vi "Update DI DAQ IO Data.vi"(8 "error in (no error)":errorcluster, 9 "DIO in":bool[](array[boolean]), 10 "DIO ClusterArray":T2[](array[typedef]), 11 "dCVT DAQDict":T1) -> (0 "error out":errorcluster, 2 "DIO ClusterArray out":T2[](array[typedef]), 3 "dCVT DAQDict out":T1)   [LabVIEW 2020, in "DAQDict.lvlib"]
uses:
  DAQDict.lvlib
  support/IO Task--cluster.ctl
  support/IO Task Dict Node--cluster.ctl
  support/IONameNode--cluster.ctl
  support/DIO ClusterArray Element--cluster.ctl
  <vilib>/TELLC/Dynamic CVT API/TD Dynamic CVT DVR--ref.ctl
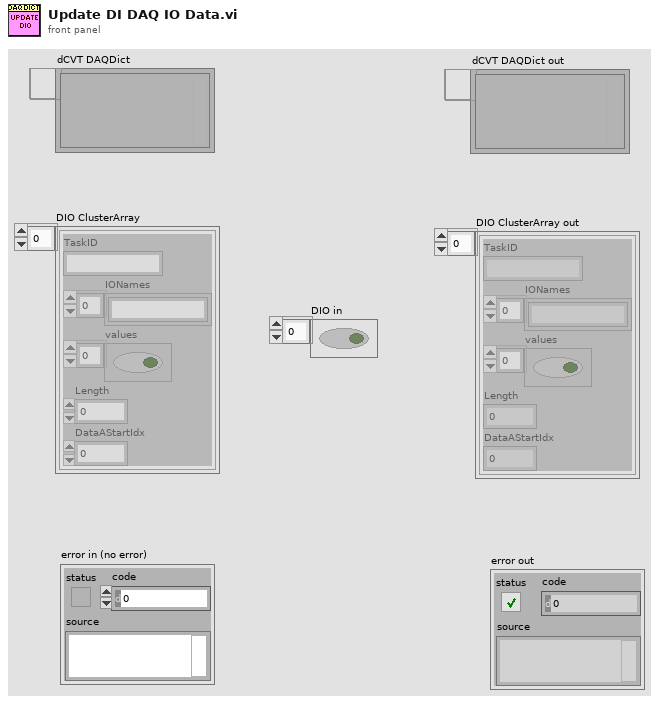
[diagram p1: front panel]
types:
  T1 = typedef "TD Dynamic CVT DVR--ref.ctl" = refnum<data-value>
  T2 = typedef "DIO ClusterArray Element--cluster.ctl" = cluster{"TaskID":string, "IONames":string[], "values":bool[], "Length":i32, "DataAStartIdx":i32}
  T3 = typedef "IO Task Dict Node--cluster.ctl" = cluster{"IO Type":enum16{"N/A", "DI", "DO"}, "IONames":string[], "values":bool[], "IO Task":T4}
  T4 = typedef "IO Task--cluster.ctl" = cluster{"IO Type":enum16{"N/A", "DI", "DO"}, "TaskID":string, "IONames":string[], "ChPath":string[], "Task Ref":refnum<k21>}
  T5 = typedef "IONameNode--cluster.ctl" = cluster{"IOName":string, "value":bool, "IO Type":enum16{"N/A", "DI", "DO"}, "TaskID":string, "data Idx":i32}
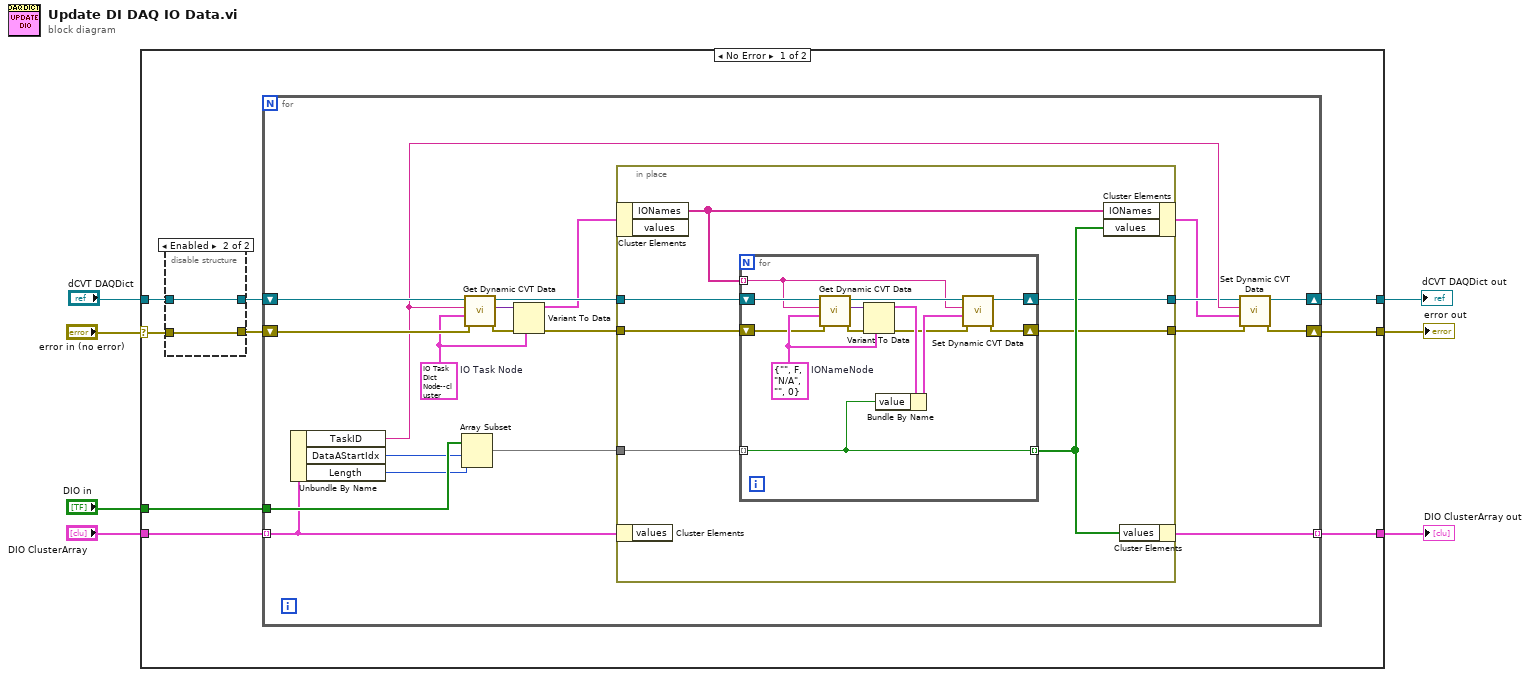
[diagram p0: block diagram]
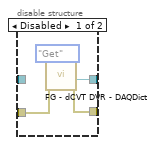
[diagram p2: hidden frame]
diagram:
  n1 = case shown="No Error" "error in (no error)" {
    selector: "error in (no error)" -> [w10 w65]
    tunnel: "DIO ClusterArray" -> [w15 w64]
    tunnel: "DIO in" -> [w14 _]
    tunnel: [w13 w64] -> w5
    tunnel: [w12 w65] -> w4
    tunnel: "dCVT DAQDict" -> [w9 w63]
    tunnel: [w8 w63] -> w1
    frame No Error {
      n2 = disable-structure shown="Enabled" {
        disable-tunnel: [w19 w22] -> w16
        disable-tunnel: [w18 w21] -> w11
        disable-tunnel: w10 -> [w17 w21]
        disable-tunnel: w9 -> [_ w22]
        frame Disabled {
          n3 = call "FG - dCVT DVR - DAQDict.vi"("error in (no error)"=w17, "Action (Get)"=enum16{"Init", "Get", "Set"}."Get") -> ("dCVT DAQDict out"=w19:T1, "error out"=w18:errorcluster)  [unwired: 7 in]
        }
        frame Enabled {
        }
      }
      n4 = for {
        shift-right: [w40] -> w8
        shift-left: w16 -> [w42]
        shift-right: [w39] -> w12
        shift-left: w11 -> [w41]
        tunnel: w15 -> [w37] mode=indexing
        tunnel: w14 -> [w38]
        tunnel: [w33] -> w13 mode=indexing
        w29 = T3 {"IO Type"=enum."N/A", "IONames"=[], "values"=[], "IO Task"={"IO Type"=enum."N/A", "TaskID"="", "IONames"=[], "ChPath"=[], "Task Ref"=""}}  # IO Task Node
        n5 = Unbundle By Name(w37) -> ("TaskID"=w36:string, "DataAStartIdx"=w35:i32, "Length"=w34:i32)
        n6 = Array Subset(array=w38, index=w35, length=w34) -> (w27:bool[])
        n7 = call <vilib>:"Get Dynamic CVT Data.vi"("error in (no error)"=w41, "default value (empty variant)"=w29, "DataName"=w36, "dCVT DVR"=w42) -> ("error out"=w31:errorcluster, "value"=w32:variant, "dCVT DVR out"=w30:T1)  [unwired: 4 in, 1 out]
        n8 = Variant To Data(error in=w31, type=w29, Variant=w32) -> (data=w28:T3, error out=w26:errorcluster)
        n9 = in-place {
          in-place-border: w30 -> [w49]
          in-place-border: w27 -> [w47]
          in-place-border: w26 -> [w46]
          in-place-border: [w44] -> w25
          in-place-border: [w43] -> w24
          n10 = in-place-cluster #1(w28) -> ("IONames"=w48:string[])  [unwired: 1 out]
          n11 = in-place-cluster #2(w37) -> ()  [unwired: 1 out]
          n12 = for {
            tunnel: w48 -> [w55] mode=indexing
            shift-right: [w53] -> w44
            shift-left: w49 -> [w62]
            tunnel: w47 -> [w52] mode=indexing
            shift-right: [w51] -> w43
            shift-left: w46 -> [w50]
            tunnel: [w52] -> w45 mode=indexing
            w59 = T5 {"IOName"="", "value"=FALSE, "IO Type"=enum."N/A", "TaskID"="", "data Idx"=0}  # IONameNode
            n13 = call <vilib>:"Get Dynamic CVT Data.vi"("error in (no error)"=w50, "default value (empty variant)"=w59, "DataName"=w55, "dCVT DVR"=w62) -> ("error out"=w60:errorcluster, "value"=w61:variant, "dCVT DVR out"=w57:T1)  [unwired: 4 in, 1 out]
            n14 = Variant To Data(error in=w60, type=w59, Variant=w61) -> (data=w58:T5, error out=w54:errorcluster)
            n15 = Bundle By Name(cluster=w58, "value"=w52) -> (w56:T5)
            n16 = call <vilib>:"Set Dynamic CVT Data.vi"("error in (no error)"=w54, "value"=w56, "DataName"=w55, "dCVT DVR"=w57) -> ("error out"=w51:errorcluster, "dCVT DVR out"=w53:T1)  [unwired: 5 in, 1 out]
          }
          n17 = in-place-cluster #1("IONames"=w48, "values"=w45) -> (w23:T3)
          n18 = in-place-cluster #2("values"=w45) -> (w33:T2)
        }
        n19 = call <vilib>:"Set Dynamic CVT Data.vi"("error in (no error)"=w24, "value"=w23, "DataName"=w36, "dCVT DVR"=w25) -> ("error out"=w39:errorcluster, "dCVT DVR out"=w40:T1)  [unwired: 5 in, 1 out]
      }
    }
    frame Error {
    }
  }
  "DIO ClusterArray out" <- w5
  "error out" <- w4
  "dCVT DAQDict out" <- w1
